vi "Quick Start - Simple - Get All Units.vi"() -> ()   [LabVIEW 2020]
uses:
  Nominal Client/Nominal Client.lvclass/Nominal Client.ctl
  f0812496-c75d-44b0-8270-75918c1a52ee.vi
  Nominal Client/private_data.set.vi
  <vilib>/Utility/file.llb/Application Directory.vi
  <vilib>/Utility/error.llb/Error Cluster From Error Code.vi
  submodules/reqwest-labview/lv-src/reqwest/create.vi
  <vilib>/JDP Science/JSONtext/Pretty Print.vi
  Nominal Client/Nominal Client.lvclass
  nominal types/workspace/workspace.lvclass
  submodules/reqwest-labview/lv-src/reqwest/reqwest.lvclass
panel:
  out "Response":string
  # "See block diragram for usage instructions"
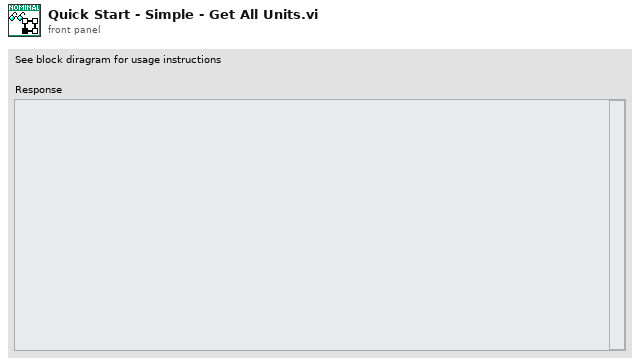
[diagram p1: front panel]
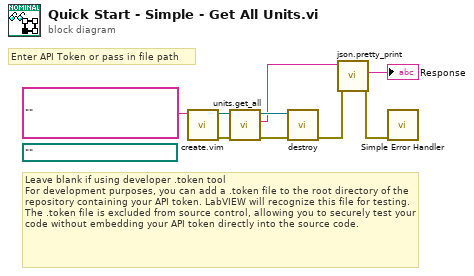
[diagram p0: block diagram]
diagram:
  (unwired) path ""
  # "Leave blank if using developer .token tool\nFor development purposes, you can add a .token file to the root directory of the repository containing your API token. LabVIEW will recognize this file for testing. The .token file is excluded from source control, allowing you to securely test your code without embedding your API token directly into the source code."
  # "Enter API Token or pass in file path"
  n1 = call "create.vim"("API Token (string or path)"="" ("API Token")) -> ("error out"=w8:errorcluster, "Nominal Client"=w9:refnum<class "Nominal Client.lvclass">)  [unwired: 9 in]
  n2 = call "units.get_all.vi"("error in"=w8, "Nominal Client in"=w9) -> ("error out"=w6:errorcluster, "Response body"=w5:string, "Nominal Client out"=w7:refnum<class "Nominal Client.lvclass">)  [unwired: 7 in]
  n3 = call "destroy.vi"("error in"=w6, "Nominal Client"=w7) -> ("error out"=w3:errorcluster)  [unwired: 9 in]
  n4 = call "json.pretty_print.vi"("error in"=w3, "JSON in"=w5) -> ("error out"=w2:errorcluster, "Pretty JSON Out"=→"Response":string)  [unwired: 8 in]
  n5 = call <vilib>:"Simple Error Handler.vi"("error in (no error)"=w2) -> ()  [unwired: 4 in, 5 out]
